vi "FPGA Clock Decimator.vi"(7 "Reset":bool, 9 "Idle State":enum16{"Idle Low", "Idle High"}(ring), 10 "Decimation Factor":u16, 11 "Clock In":bool) -> (3 "Clock Out":bool)   [LabVIEW 2014]
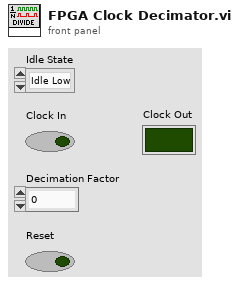
[diagram p1: front panel]
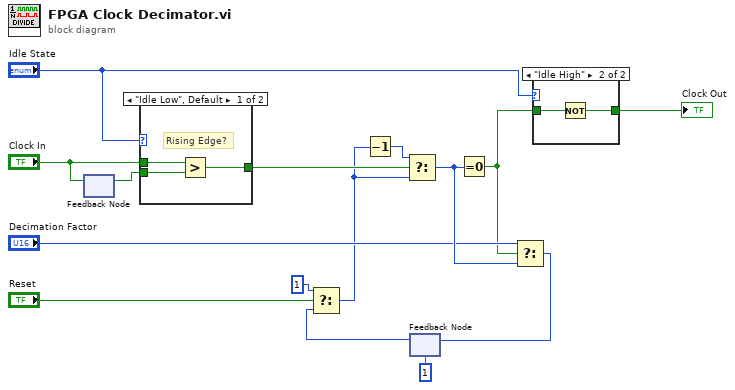
[diagram p0: block diagram]
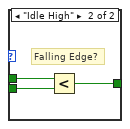
[diagram p3: hidden frame]
diagram:
  n1 = feedback-in #1("Clock In") -> ()
  n2 = feedback #1() -> (w10:bool)  [unwired: 1 in]
  n3 = case shown="\"Idle Low\", Default" "Idle State" {
    tunnel: "Clock In" -> [w18 w20]
    tunnel: w10 -> [w17 w19]
    tunnel: [w16 w21] -> w14
    frame "Idle Low", Default {
      # "Rising Edge?"
      n4 = Greater?(x=w18, y=w17) -> (0:w16:bool)
    }
    frame "Idle High" {
      # "Falling Edge?"
      n5 = Less?(x=w20, y=w19) -> (x < y?=w21:bool)
    }
  }
  n6 = feedback #2(u16 1) -> (w2:u16)
  n7 = Select(t=u16 1, s="Reset", f=w2) -> (s? t:f=w1:u16)
  n8 = Decrement(x=w1) -> (x-1=w15:u16)
  n9 = Select(t=w15, s=w14, f=w1) -> (s? t:f=w9:u16)
  n10 = Equal To 0?(x=w9) -> (x = 0?=w6:bool)
  n11 = Select(t="Decimation Factor", s=w6, f=w9) -> (s? t:f=w3:u16)
  n12 = feedback-in #2(w3) -> ()
  n13 = case shown="\"Idle High\"" "Idle State" {
    tunnel: w6 -> [w22 w24]
    tunnel: [w22 w23] -> w12
    frame "Idle Low", Default {
    }
    frame "Idle High" {
      n14 = Not(x=w24) -> (.not. x?=w23:bool)
    }
  }
  "Clock Out" <- w12
